vi "GetTopicNode_etc.vi"(4 "Node":cluster{"name":string, "Port":u16}, 5 "Definitions":T3={"Topic"="/robot/head/command_head_nod", "Type"="std_msgs/Bool", "Action"=enum."Publisher", "Update (ms)"=1, "queue size"=1}) -> (2 "ROS":T1={"topic port"=0, "Node"="", "topic"="", "type"="", "node port"=0, "error "={"status"=FALSE, "code"=0, "source"=""}, "Direction"=enum."Node", "Update (ms)"=1, "FIFO size"=1})   [LabVIEW 2014]
doc: "Gets the node for a topic and checks whether it is running and has an HTML page"
uses:
  <userlib>/ROS for LabVIEW Software.lnk/ROS/Code/Console/Servers/ServerSubs/TopicDef.ctl
  <userlib>/ROS for LabVIEW Software.lnk/ROS/Code/SubVIs/_ROSDirection.ctl
  <userlib>/ROS for LabVIEW Software.lnk/ROS/Code/SubVIs/_ROSControl.ctl
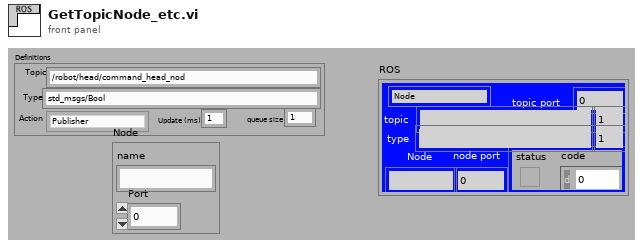
[diagram p1: front panel]
types:
  T1 = typedef "_ROSControl.ctl" = cluster{"topic port":u16, "Node":string, "topic":string, "type":string, "node port":u16, "error ":errorcluster, "Direction":T2, "Update (ms)":u16, "FIFO size":u16}
  T2 = typedef "_ROSDirection.ctl" = enum16{"Node", "Publisher", "Subscriber", "ServiceClient", "ServiceProvider"}
  T3 = typedef "TopicDef.ctl" = cluster{"Topic":string, "Type":string, "Action":T2, "Update (ms)":u16, "queue size":u16}
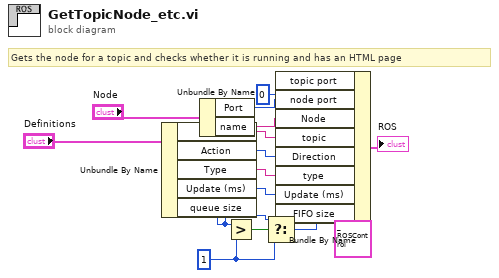
[diagram p0: block diagram]
diagram:
  w1 = u16 1 ("f")
  # "Gets the node for a topic and checks whether it is running and has an HTML page"
  n1 = Unbundle By Name("Definitions") -> ("Topic"=w11:string, "Action"=w10:T2, "Type"=w9:string, "Update (ms)"=w8:u16, "queue size"=w2:u16)
  n2 = Unbundle By Name("Node") -> ("Port"=w13:u16, "name"=w12:string)
  n3 = Greater?(x=w2, y=w1) -> (0:w7:bool)
  n4 = Select(t=w2, s=w7, f=w1) -> (s? t:f=w6:u16)
  n5 = Bundle By Name(cluster=T1 {"topic port"=0, "Node"="", "topic"="", "type"="", "node port"=0, "error "={"status"=FALSE, "code"=0, "source"=""}, "Direction"=enum."Node", "Update (ms)"=1, "FIFO size"=1} ("ROS"), "topic port"=u16 0, "node port"=w13, "Node"=w12, "topic"=w11, "Direction"=w10, "type"=w9, "Update (ms)"=w8, "FIFO size"=w6) -> (→"ROS":T1)
